vi "ROI Apply.vi"(8 "error in (no error)":errorcluster, 11 "ROIed Video Frame in":refnum<class "ROIed Video Frame.lvclass">) -> (0 "error out":errorcluster, 3 "ROIed Video Frame out":refnum<class "ROIed Video Frame.lvclass">)   [LabVIEW 2018, in "ROIed Video Frame.lvclass"]
uses:
  ROIed Video Frame.lvclass
  ROIed Video Frame.lvclass/ROIed Video Frame.ctl
  <vilib>/vision/NI_Vision_Development_Module.lvlib
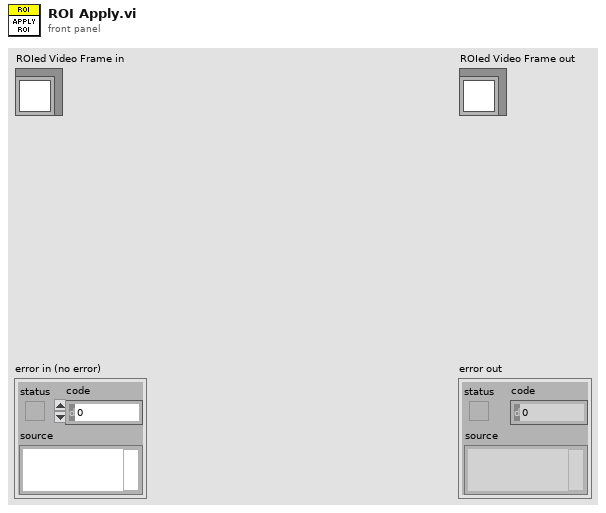
[diagram p1: front panel]
types:
  T1 = typedef "ROI Descriptor" = cluster{"Global Rectangle":i32[], "Contours":cluster{"ID":enum32{"External", "Internal"}, "Type":u32, "Coordinates":i32[]}[]}
  T2 = typedef "IMAQ Image.ctl" = refnum<image>
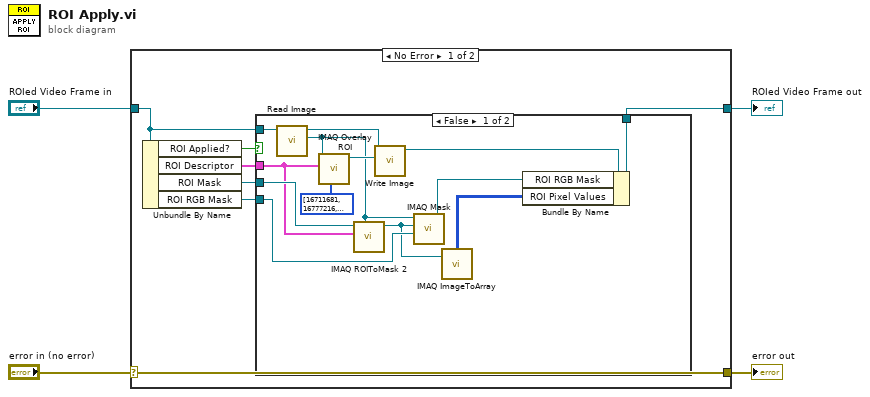
[diagram p0: block diagram]
diagram:
  n1 = case shown="No Error" "error in (no error)" {
    selector: "error in (no error)" -> [w11 w27]
    tunnel: [w11 w27] -> w3
    tunnel: [w6 w26] -> w1
    tunnel: "ROIed Video Frame in" -> [w5 w26]
    frame No Error {
      n2 = Unbundle By Name(w5) -> ("ROI Applied?"=w10:bool, "ROI Descriptor"=w9:T1, "ROI Mask"=w8:T2, "ROI RGB Mask"=w7:T2)
      n3 = case shown="False" w10 {
        tunnel: w9 -> [w21 _]
        tunnel: w8 -> [w22 _]
        tunnel: w5 -> [w24 w25]
        tunnel: w7 -> [w17 _]
        tunnel: [w12 w25] -> w6
        frame False {
          n4 = call-dynamic "Read Image.vi"("Video Frame in"=w24) -> ("Image"=w18:T2, "Video Frame out"=w20:refnum<class "ROIed Video Frame.lvclass">)  [unwired: 8 in, 1 out]
          n5 = call "IMAQ Overlay ROI"("Colors (Green)"=u32[] [16711681, 16777216, 16777216, 0, 16777216, 16777216, 16777216] ("Point Symbol"), "ROI Descriptor"=w21, "Image"=w18) -> ("Image Out"=w19:T2)  [unwired: 7 in, 1 out]
          n6 = call "IMAQ ROIToMask 2"("Image Model"=w18, "ROI Descriptor"=w21, "Image"=w22) -> ("Image Out"=w14:T2)  [unwired: 6 in, 2 out]
          n7 = call-dynamic "Write Image.vi"("Image"=w19, "Video Frame in"=w20) -> ("Video Frame out"=w16:refnum<class "ROIed Video Frame.lvclass">)  [unwired: 8 in, 1 out]
          n8 = call "IMAQ Mask"("Image Dst"=w17, "Image Mask"=w14, "Image Src"=w18) -> ("Image Dst Out"=w15:T2)  [unwired: 2 in, 1 out]
          n9 = call "IMAQ ImageToArray"("Image"=w14) -> ("Image Pixels (U8)"=w13:u8[][])  [unwired: 3 in, 4 out]
          n10 = Bundle By Name(cluster=w16, "ROI RGB Mask"=w15, "ROI Pixel Values"=w13) -> (w12:refnum<class "ROIed Video Frame.lvclass">)
        }
        frame True {
        }
      }
    }
    frame Error {
    }
  }
  "error out" <- w3
  "ROIed Video Frame out" <- w1
